vi "SandDropInit.vi"(10 "Height":i32=20, 11 "Width":i32=26) -> (3 "Array":string[][](array[string]))   [LabVIEW 2013]
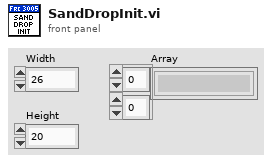
[diagram p1: front panel]
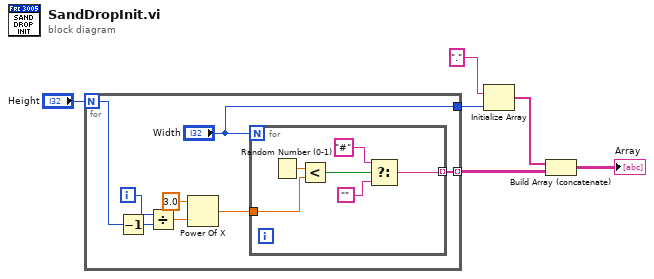
[diagram p0: block diagram]
diagram:
  n1 = for {
    N: "Height" -> [w12]
    tunnel: [w14] -> w3 mode=indexing
    tunnel: ["Width"] -> w6
    i -> [w13]
    n2 = Decrement(x=w12) -> (x-1=w11:i32)
    n3 = Divide(x=w13, y=w11) -> (x/y=w10:dbl)
    n4 = Power Of X(1:w10, 2:3.0 ("y")) -> (0:w9:dbl)
    n5 = for {
      N: "Width" -> [_]
      tunnel: [w17] -> w14 mode=indexing
      tunnel: w9 -> [w18]
      n6 = Random Number (0-1)() -> (number: 0 to 1=w20:dbl)
      n7 = Less?(x=w20, y=w18) -> (x < y?=w16:bool)
      n8 = Select(t="#", s=w16, f="") -> (s? t:f=w17:string)
    }
  }
  n9 = Initialize Array(".", w6) -> (w4:string[])
  n10 = Build Array (concatenate)(w4, w3) -> (→"Array":string[][])
